vi "LithographyConvertUnits.vi"(8 "error in (no error)":errorcluster, 11 "AFM_Driver in":refnum<class "AFM_Driver.lvclass">) -> (0 "error out":errorcluster, 3 "AFM_Driver out":refnum<class "AFM_Driver.lvclass">)   [LabVIEW 2019, in "AFM_Driver.lvclass"]
uses:
  AFM_Driver.lvclass
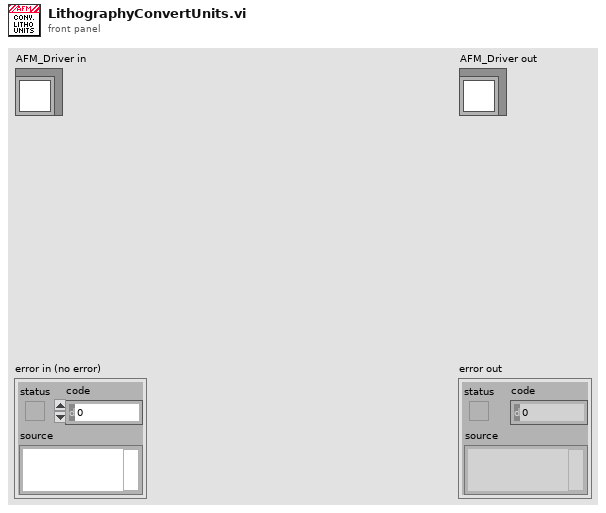
[diagram p1: front panel]
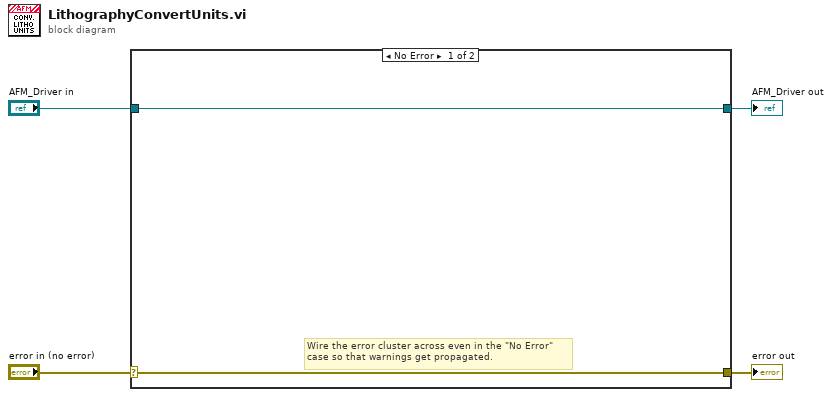
[diagram p0: block diagram]
diagram:
  n1 = case shown="No Error" "error in (no error)" {
    selector: "error in (no error)" -> [w5 w8]
    tunnel: [w5 w8] -> w3
    tunnel: [w6 w7] -> w1
    tunnel: "AFM_Driver in" -> [w6 w7]
    frame No Error {
      # "Wire the error cluster across even in the \"No Error\"\ncase so that warnings get propagated."
    }
    frame Error {
    }
  }
  "error out" <- w3
  "AFM_Driver out" <- w1
